vi "Split String.vi"(1 "Ignore Case? (false)":bool, 4 "Split Pattern":string, 6 "Input String":string) -> (2 "Split String":string[](array[string]))   [LabVIEW 2020]
doc: "Splits a string at a pattern into an array of strings.\n\n<B>Input String</B> - The string to split.\n<B>Split Pattern</B> - The regular expression to split the string at.\n<B>Ignore Case?</B> - Should case be ignored in the <B>Split Pattern</B>.\n<B>Split String</B> - The array of elements between found instances of <B>Split Pattern</B> in <B>Input String</B>."
uses:
  <vilib>/regexp/Match Regular Expression.xnode
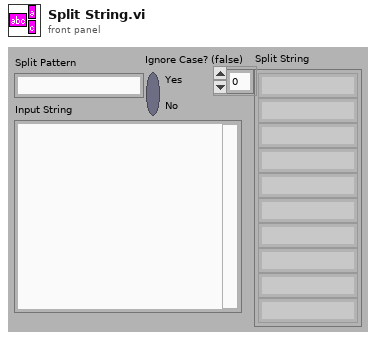
[diagram p1: front panel]
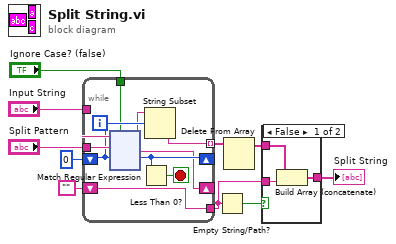
[diagram p0: block diagram]
diagram:
  n1 = while {
    tunnel: "Split Pattern" -> [w20]
    tunnel: "Input String" -> [w19]
    shift-right: [w18] -> _
    shift-left: 0 ("offset past match") -> [w16]
    tunnel: [w14] -> w7 mode=indexing
    tunnel: [w12] -> w4
    shift-right: [w13] -> _
    shift-left: "" -> [w12]
    tunnel: "Ignore Case? (false)" -> [w11]
    stop <- w17 stop-if-true
    n2 = xnode "Match Regular Expression"("input string"=w19, "regular expression"=w20, "offset (0)"=w16, "ignore case? (F)"=w11) -> ("before match"=w15:string, "after match"=w13:string, "offset past match"=w18:i32)  [unwired: 2 in, 2 out]
    n3 = Less Than 0?(x=w18) -> (x < 0?=w17:bool)
    n4 = String Subset(string=w15, offset (0)=w16) -> (substring=w14:string)  [unwired: 1 in]
  }
  n5 = Empty String/Path?(string/path=w4) -> (empty?=w3:bool)
  n6 = Delete From Array(array=w7) -> (array with subset deleted=w6:string[])  [unwired: 2 in, 1 out]
  n7 = case shown="False" w3 {
    tunnel: w6 -> [w137 w138]
    tunnel: [w136 w138] -> w5
    tunnel: w4 -> [w135 _]
    frame False {
      n8 = Build Array (concatenate)(w137, w135) -> (w136:string[])
    }
    frame True {
    }
  }
  "Split String" <- w5
